vi "Untitled 1.vi"() -> ()   [LabVIEW 2016]
panel:
  out "Dist Out":dbl
  in  "Target in":T1
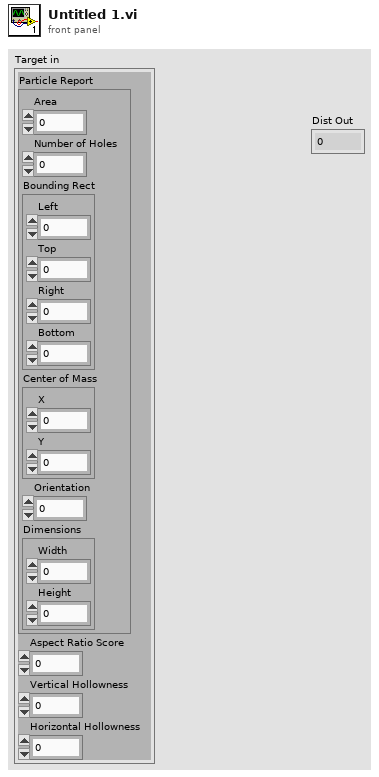
[diagram p1: front panel]
types:
  T1 = cluster{"Particle Report":cluster{"Area":dbl, "Number of Holes":dbl, "Bounding Rect":cluster{"Left":dbl, "Top":dbl, "Right":dbl, "Bottom":dbl}, "Center of Mass":cluster{"X":dbl, "Y":dbl}, "Orientation":dbl, "Dimensions":cluster{"Width":dbl, "Height":dbl}}, "Aspect Ratio Score":dbl, "Vertical Hollowness":dbl, "Horizontal Hollowness":dbl}
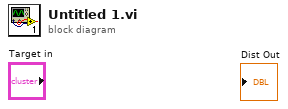
[diagram p0: block diagram]
diagram:
